vi "Read Settings by ID.vi"(8 "error in (no error)":errorcluster, 10 "Settings ID":string, 11 "Configuration Session in":refnum<class "Configuration Session.lvclass">) -> (0 "error out":errorcluster, 1 "values":cluster{"key":string, "value":string}[](array[cluster]), 3 "Configuration Session out":refnum<class "Configuration Session.lvclass">, 4 "found?":bool)   [LabVIEW 2017, in "DSF Core.lvlib" / "Configuration Session.lvclass"]
doc: "Reads a value associated with a key in a specified section from the configuration data identified by <B>dsf refnum</B>. If the key does not exist, the VI returns the default value. This VI supports multibyte characters in strings. Wire data to the <B>default value</B> input to determine the polymorphic instance to use or manually select the instance."
uses:
  Configuration Session.lvclass
  Configuration Session.lvclass/Configuration Session.ctl
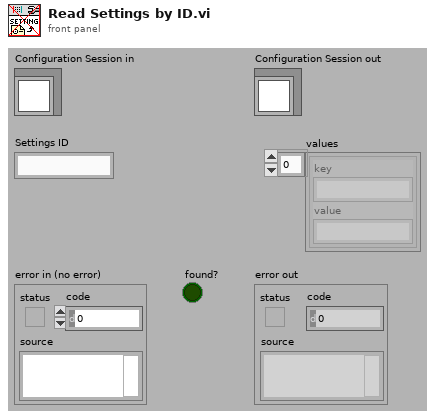
[diagram p1: front panel]
types:
  T1 = typedef "DSF Core.lvlib/Configuration Session.lvclass/DSF Config Data Ref.ctl" = refnum<data-value>
  T2 = typedef "DSF Core.lvlib/Configuration Session.lvclass/DSF Config Data.ctl" = cluster{"dsf configuration":T3, "path":path, "dirty":bool}
  T3 = typedef "DSF Core.lvlib/Configuration Session.lvclass/Internal DSF Configuration.ctl" = cluster{"dsfversion":T4, "version":T4, "plugins":T5[], "groups":T10[], "transfers":T12[], "channels":T14[], "settings":T16[], "framework configuration":T18}
  T4 = typedef "DSF Core.lvlib/DSF Version Info.ctl" = cluster{"major":u32, "minor":u32, "fix":u32, "build":string}
  T5 = typedef "DSF Core.lvlib/Configuration Session.lvclass/Internal DSF Plugin with ID.ctl" = cluster{"id":string, "values":T6}
  T6 = typedef "DSF Core.lvlib/Configuration Session.lvclass/Internal DSF Plugin Info.ctl" = cluster{"components":string[], "timing":T7, "group ids":string[], "settings id":string, "threads":T8[]}
  T7 = typedef "DSF Core.lvlib/DSF Timing Info.ctl" = cluster{"priority":u64, "decimation":u64, "offset":u64}
  T8 = typedef "DSF Core.lvlib/DSF Engine Plugin Thread Configuration.ctl" = cluster{"processor":i32, "priority offset":i16, "settings":T9}
  T9 = typedef "DSF Core.lvlib/DSF Settings Info.ctl" = cluster{"component":string, "name":string, "values":cluster{"key":string, "value":string}[]}[]
  T10 = typedef "DSF Core.lvlib/Configuration Session.lvclass/Internal DSF Group with ID.ctl" = cluster{"id":string, "values":T11}
  T11 = typedef "DSF Core.lvlib/Configuration Session.lvclass/Internal DSF Group Info.ctl" = cluster{"direction":i32, "timing":T7, "transfer ids":string[], "settings id":string, "thread":i32, "timeout behavior":u8}
  T12 = typedef "DSF Core.lvlib/Configuration Session.lvclass/Internal DSF Transfer with ID.ctl" = cluster{"id":string, "values":T13}
  T13 = typedef "DSF Core.lvlib/Configuration Session.lvclass/Internal DSF Transfer Info.ctl" = cluster{"byte order":i32, "channel ids":string[], "settings id":string}
  T14 = typedef "DSF Core.lvlib/Configuration Session.lvclass/Internal DSF Channel with ID.ctl" = cluster{"id":string, "values":T15}
  T15 = typedef "DSF Core.lvlib/Configuration Session.lvclass/Internal DSF Channel Info.ctl" = cluster{"string buffer offset":u64, "string data type":i32, "engine data type":i32, "settings id":string, "units":string}
  T16 = typedef "DSF Core.lvlib/Configuration Session.lvclass/Internal DSF Settings with ID.ctl" = cluster{"id":string, "values":T17}
  T17 = typedef "DSF Core.lvlib/Configuration Session.lvclass/Internal DSF Settings Info.ctl" = cluster{"key":string, "value":string}[]
  T18 = typedef "DSF Core.lvlib/DSF Engine Framework Configuration.ctl" = cluster{"plugins":T19[]}
  T19 = typedef "DSF Core.lvlib/DSF Engine Plugin Configuration.ctl" = cluster{"name":string, "components":string[], "cycle timing":T7, "threads":T8[], "transfer groups":T20[], "settings":T9}
  T20 = typedef "DSF Core.lvlib/DSF Engine Transfer Group Configuration.ctl" = cluster{"name":string, "direction":T21, "cycle timing":T7, "thread index":u8, "settings":T9, "transfers":T22[], "timeout behavior":T26, "convert buffers":bool}
  T21 = typedef "DSF Core.lvlib/DSF Direction.ctl" = enum8{"Tx", "Rx"}
  T22 = typedef "DSF Core.lvlib/DSF Engine Transfer Configuration.ctl" = cluster{"name":string, "string byte order":T23, "settings":T9, "channels":T24[]}
  T23 = typedef "DSF Core.lvlib/DSF Byte Order.ctl" = enum8{"big-endian", "little-endian"}
  T24 = typedef "DSF Core.lvlib/DSF Engine Channel Configuration.ctl" = cluster{"string offset":u64, "name":string, "units":string, "engine data type":T25, "string data type":T25, "settings":T9}
  T25 = typedef "DSF Core.lvlib/DSF Data Type.ctl" = enum8{"Bool", "SGL", "DBL", "I8", "I16", "I32", "I64", "U8", "U16", "U32", "U64"}
  T26 = typedef "DSF Core.lvlib/DSF Timeout Behavior.ctl" = enum8{"Increment Late Count", "Throw Error"}
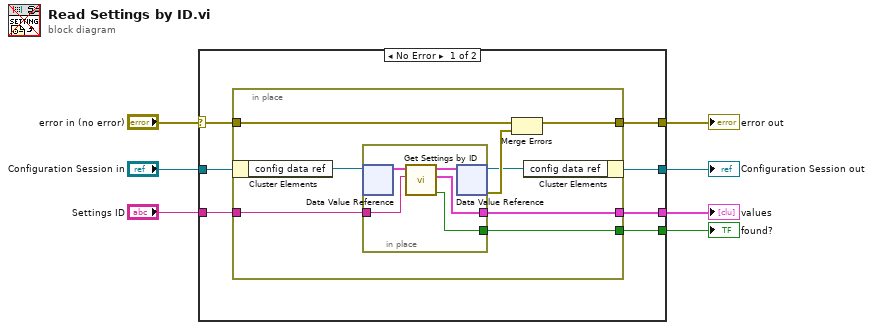
[diagram p0: block diagram]
diagram:
  n1 = case shown="No Error" "error in (no error)" {
    selector: "error in (no error)" -> [w8 w29]
    tunnel: "Settings ID" -> [w14 _]
    tunnel: [w13 _] -> w6
    tunnel: [w12 _] -> w5
    tunnel: "Configuration Session in" -> [w11 w28]
    tunnel: [w10 w29] -> w3
    tunnel: [w9 w28] -> w2
    frame No Error {
      n2 = in-place {
        in-place-border: w14 -> [w22]
        in-place-border: [w21] -> w13
        in-place-border: [w20] -> w12
        in-place-border: w8 -> [w17]
        in-place-border: [w16] -> w10
        n3 = in-place-cluster #1(w11) -> ("config data ref"=w19:T1)
        n4 = in-place {
          in-place-border: w22 -> [w27]
          in-place-border: [w26] -> w21
          in-place-border: [w25] -> w20
          n5 = in-place-dvr #2(w19) -> (w24:T2)  [unwired: 1 out]
          n6 = call "Get Settings by ID.vi"("id"=w27, "DSF Configuration in"=w24) -> ("exists?"=w25:bool, "values"=w26:cluster{"key":string, "value":string}[], "DSF Configuration out"=w23:T2)  [unwired: 6 in, 1 out]
          n7 = in-place-dvr #2(w23) -> (w15:T1, w18:errorcluster)
        }
        n8 = Merge Errors(w17, w18) -> (w16:errorcluster)
        n9 = in-place-cluster #1("config data ref"=w15) -> (w9:refnum<class "Configuration Session.lvclass">)
      }
    }
    frame Error {
    }
  }
  "error out" <- w3
  "found?" <- w5
  "values" <- w6
  "Configuration Session out" <- w2
